vi "GEOM_CorrectionAddition_dataonly.vi"(8 "ini shift":u32, 9 "iniX":u32, 10 "sorted amplifiers":T1[](array[typedef]) {"fliped" items=["none", "horizontal", "vertical"]; "type" items=["LL", "LR", "UL", "UR"]}) -> (0 "out shift":u32, 1 "out x":u32, 2 "amplifiers out":T1[](array[typedef]) {"fliped" items=["none", "horizontal", "vertical"]; "type" items=["LL", "LR", "UL", "UR"]})   [LabVIEW 2016]
uses:
  GEOM_Amplifier.ctl
  GEOM_AmpType.ctl
  GEOM_ROI.ctl
  GEOM_Coords.ctl
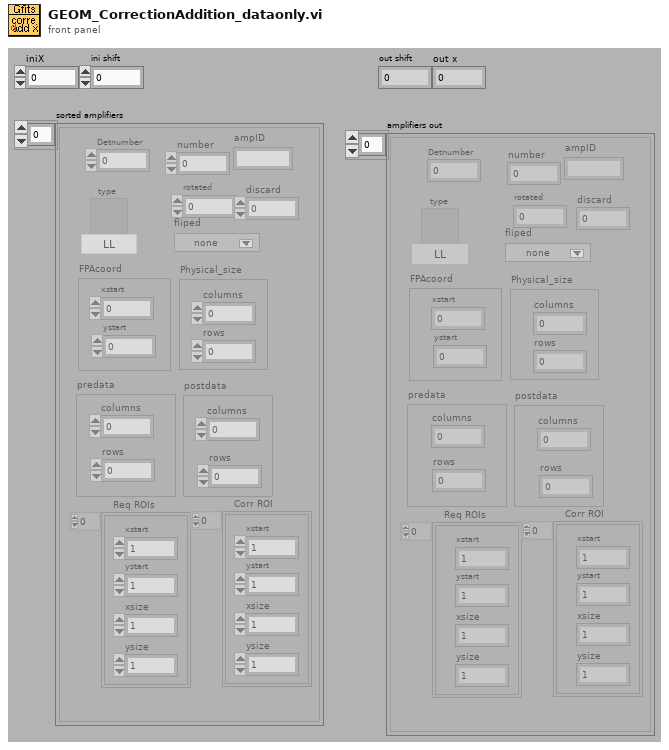
[diagram p1: front panel]
types:
  T1 = typedef "GEOM_Amplifier.ctl" = cluster{"number":i32, "type":T2, "rotated":i16, "fliped":u16, "FPAcoord":cluster{"xstart":i32, "ystart":i32}, "Physical_size":cluster{"columns":i32, "rows":i32}, "predata":cluster{"columns":i32, "rows":i32}, "postdata":cluster{"columns":i32, "rows":i32}, "Req ROIs":T3, "Corr ROI":T3, "Detnumber":i32, "ampID":string, "discard":i32}
  T2 = typedef "GEOM_AmpType.ctl" = u16
  T3 = typedef "GEOM_ROI.ctl" = T4[]
  T4 = typedef "GEOM_Coords.ctl" = cluster{"xstart":u32, "ystart":u32, "xsize":u32, "ysize":u32}
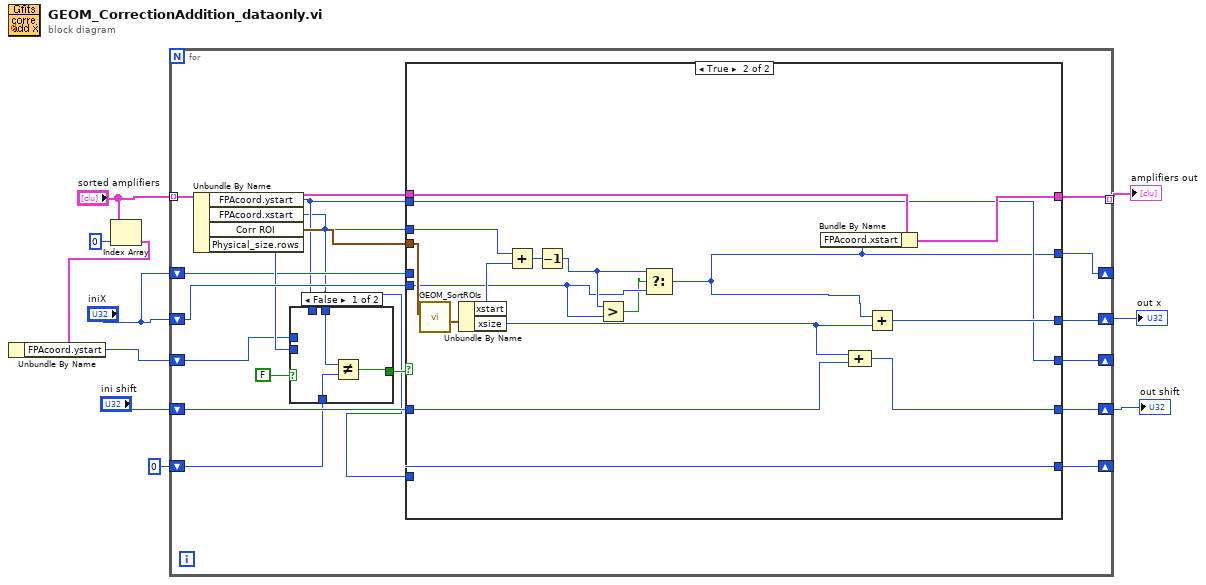
[diagram p0: block diagram]
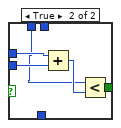
[diagram p2: hidden frame]
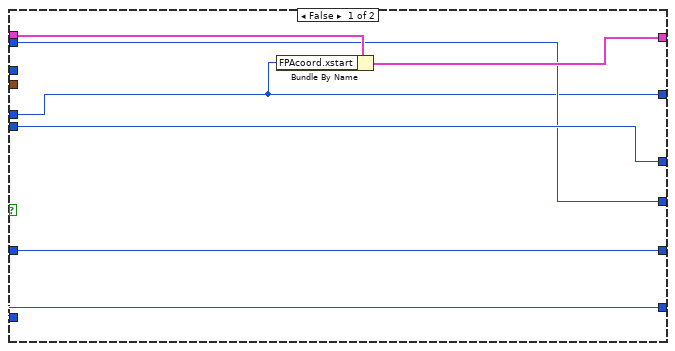
[diagram p3: hidden frame]
diagram:
  n1 = Index Array(array="sorted amplifiers", index=0) -> (element=w3:T1)
  n2 = Unbundle By Name(w3) -> ("FPAcoord.ystart"=w2:i32)
  n3 = for {
    tunnel: "sorted amplifiers" -> [w25] mode=indexing
    shift-right: [w27] -> w7
    shift-left: "iniX" -> [w22]
    tunnel: [w28] -> w10 mode=indexing
    shift-right: [w24] -> w8
    shift-left: "ini shift" -> [w23]
    shift-right: [w20] -> _
    shift-left: 0 ("ystart") -> [w12]
    shift-right: [w21] -> _
    shift-left: "iniX" -> [w17]
    shift-right: [w19] -> _
    shift-left: w2 -> [w15]
    n4 = Unbundle By Name(w25) -> ("FPAcoord.ystart"=w14:i32, "FPAcoord.xstart"=w11:i32, "Corr ROI"=w26:T3, "Physical_size.rows"=w18:i32)
    n5 = case shown="False" FALSE {
      tunnel: w18 -> [_ w36]
      tunnel: [w31 w35] -> w16
      tunnel: w15 -> [_ w33]
      tunnel: w14 -> [_ w32]
      tunnel: w11 -> [w30 _]
      tunnel: w12 -> [w29 _]
      frame False {
        n6 = Not Equal?(x=w30, y=w29) -> (x != y?=w31:bool)
      }
      frame True {
        n7 = Add(x=w33, y=w36) -> (x+y=w34:i32)
        n8 = Less?(x=w32, y=w34) -> (x < y?=w35:bool)
      }
    }
    n9 = case shown="True" w16 {
      tunnel: [w42 w60] -> w28
      tunnel: [w41 w59] -> w27
      tunnel: w26 -> [_ w58]
      tunnel: w25 -> [w43 w54]
      tunnel: [w40 w52] -> w24
      tunnel: w23 -> [w40 w51]
      tunnel: w22 -> [w41 w49]
      tunnel: w11 -> [_ w47]
      tunnel: [w37 w44] -> w21
      tunnel: w11 -> [w39 w46]
      tunnel: [w39 w46] -> w20
      tunnel: w14 -> [w38 w45]
      tunnel: [w38 w45] -> w19
      tunnel: w17 -> [w37 _]
      frame False {
        n10 = Bundle By Name(cluster=w43, "FPAcoord.xstart"=w37) -> (w42:T1)
      }
      frame True {
        n11 = call "GEOM_SortROIs.vi"("ROIs"=w58) -> ("Extreme Coords"=w57:T4)  [unwired: 10 out]
        n12 = Unbundle By Name(w57) -> ("xstart"=w56:u32, "xsize"=w53:u32)
        n13 = Add(x=w47, y=w56) -> (x+y=w55:u32)
        n14 = Decrement(x=w55) -> (x-1=w50:u32)
        n15 = Greater?(x=w50, y=w49) -> (0:w48:bool)
        n16 = Select(t=w50, s=w48, f=w49) -> (s? t:f=w44:u32)
        n17 = Bundle By Name(cluster=w54, "FPAcoord.xstart"=w44) -> (w60:T1)
        n18 = Compound Arithmetic op=ADD(w53, w51) -> (w52:u32)
        n19 = Add(x=w44, y=w53) -> (x+y=w59:u32)
      }
    }
  }
  "amplifiers out" <- w10
  "out shift" <- w8
  "out x" <- w7
